vi "Seq Dialog Check RSLinx Tag Boolean.vi"(8 "Segment Data":T3) -> (0 "Step Hisitory":string[](array[string]), 2 "Segment Data 2":T3)   [LabVIEW 2018]
uses:
  type defs/plc path and tag.ctl
  <vilib>/Platform/dataskt.llb/DataSocket Reference Type.ctl
  type defs/Sequence Info.ctl
  type defs/RSLinx Boolean Cluster.ctl
panel:
  in  "Continue on Fail for Red Rabbit":bool
  in  "timeout (ms)":i32=10000
  in  "Error No.":u16=159
  in  "Boolean":bool
  in  "Tag String":T1={"Tag Name"="S060.PXI.Signals.PlltData.SN", "Network Path"="172.15.51.1,1,0", "use opc"=FALSE, "DataSocket Reference"={"CWDSLib._DCWDataSocket"=refnum, "CWDSLib._DCWData"=refnum, "OnDataUpdated"=0, "OnStatusUpdated"=0}} {"DataSocket Reference"."OnStatusUpdated" format="%.0x"; "DataSocket Reference"."OnDataUpdated" format="%.0x"}
  out "Name":string="Pre Run Station - Glass - Vent Open"
  in  "Description":string
  in  "Save":bool
  in  "Cancel":bool
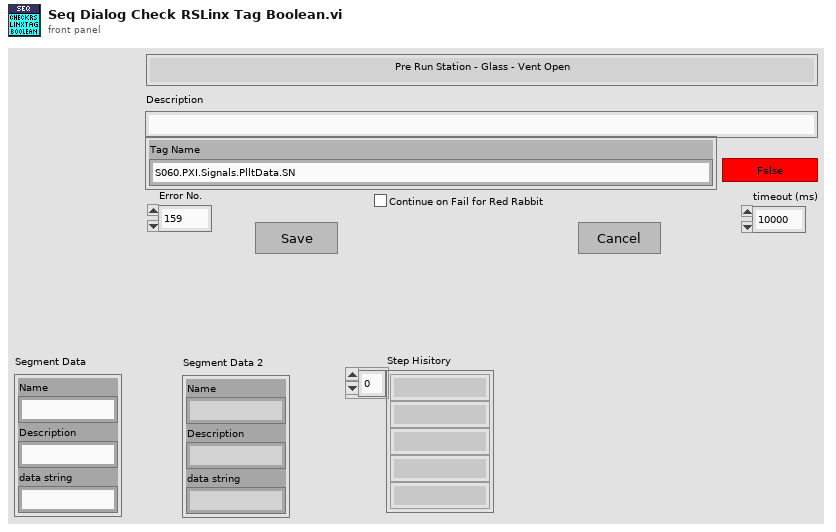
[diagram p1: front panel]
types:
  T1 = typedef "plc path and tag.ctl" = cluster{"Tag Name":string, "Network Path":string, "use opc":bool, "DataSocket Reference":T2}
  T2 = typedef "DataSocket Reference Type.ctl" = cluster{"CWDSLib._DCWDataSocket":refnum<k7>, "CWDSLib._DCWData":refnum<k7>, "OnDataUpdated":u32, "OnStatusUpdated":u32}
  T3 = typedef "Sequence Info.ctl" = cluster{"Name":string, "Description":string, "data string":string}
  T4 = typedef "RSLinx Boolean Cluster.ctl" = cluster{"Data Boolean":bool, "PLC Path and Tag":T1, "Error No.":u16, "timeout (ms)":i32, "Continue on Fail for Red-Rabbit":bool}
  T5 = cluster{"Segment Data":T3, "Old Data":string, "New Data":string, "RSLinx String Cluster":T4}
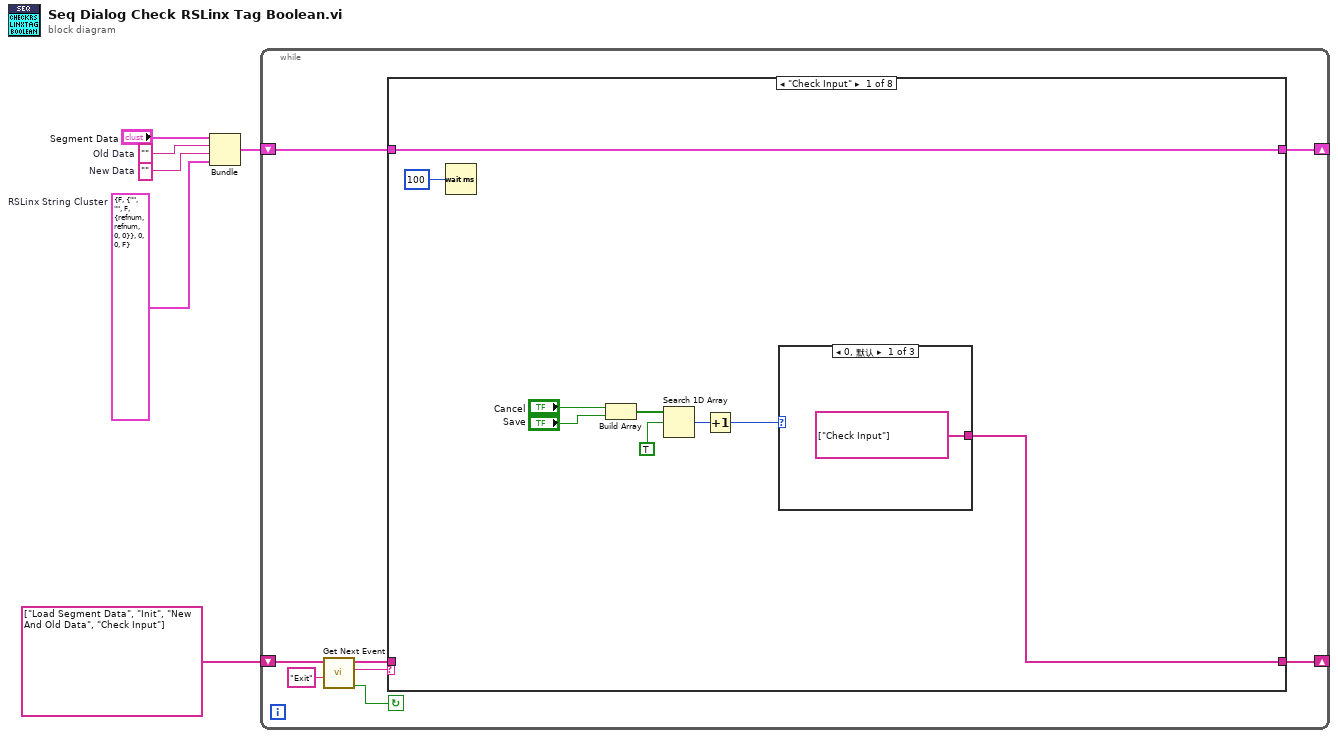
[diagram p0: block diagram]
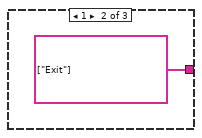
[diagram p2: hidden frame]
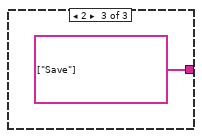
[diagram p3: hidden frame]
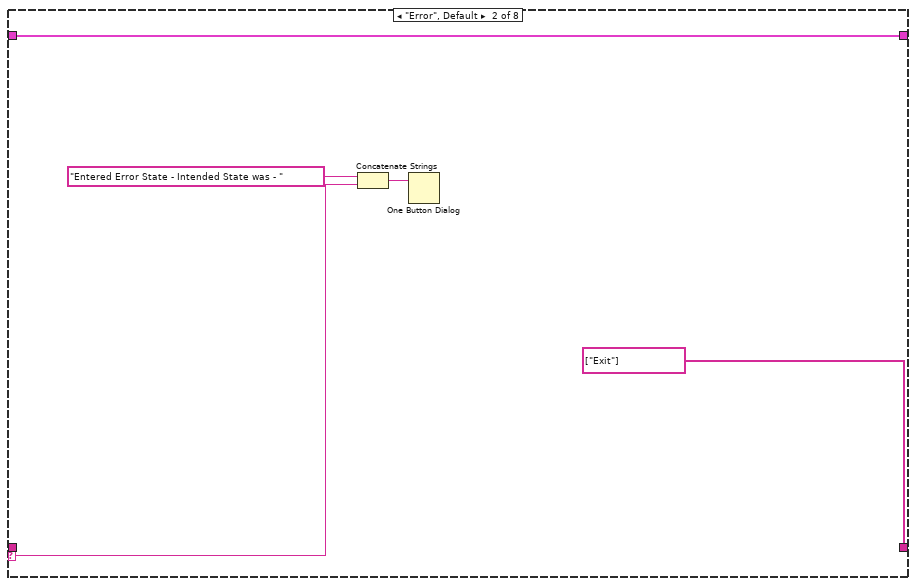
[diagram p4: hidden frame]
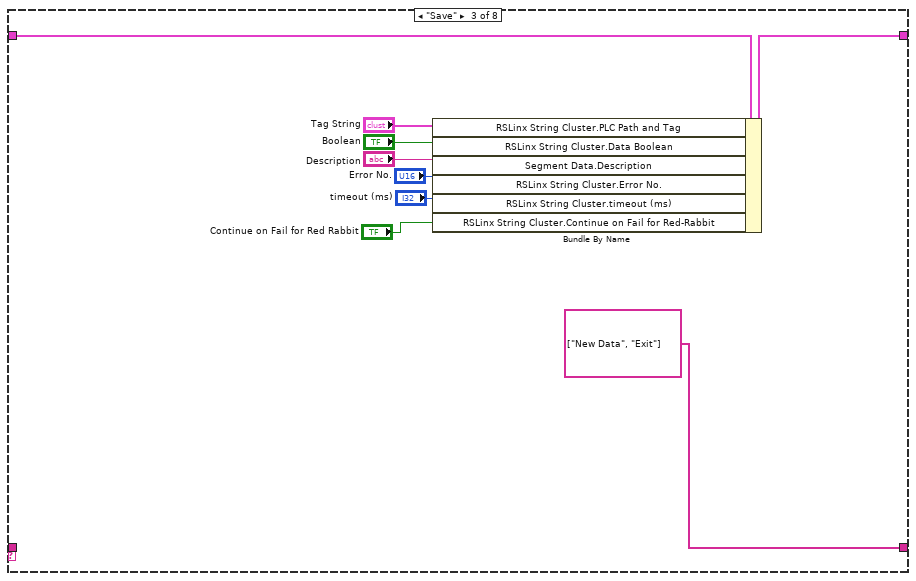
[diagram p5: hidden frame]
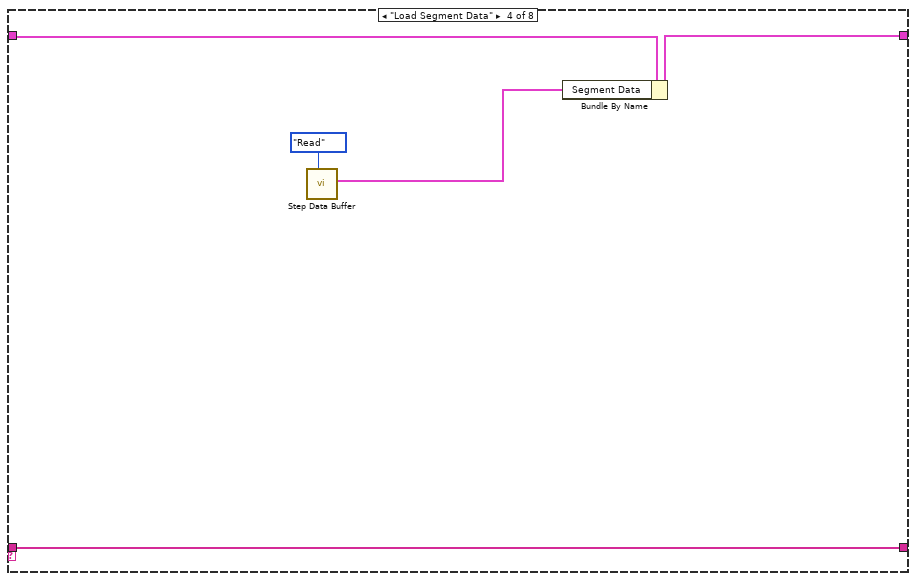
[diagram p6: hidden frame]
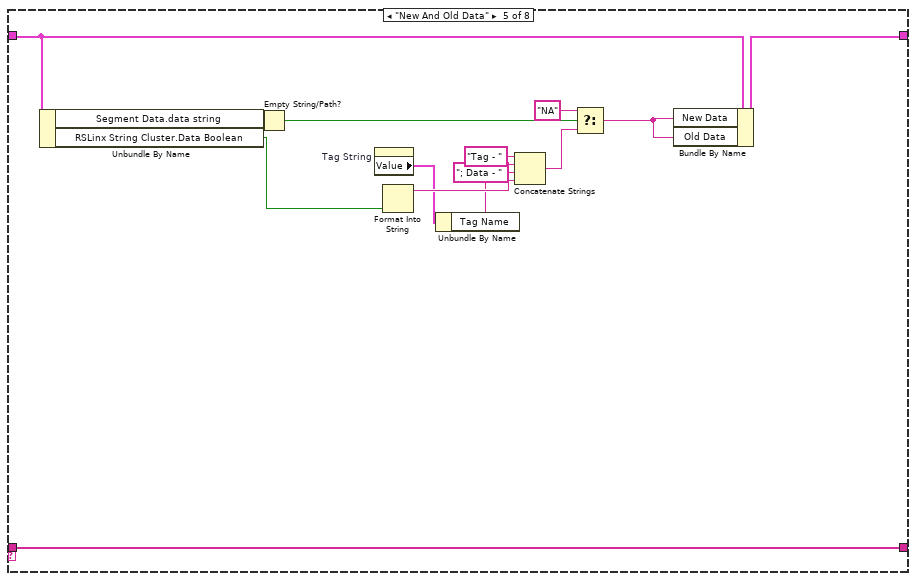
[diagram p7: hidden frame]
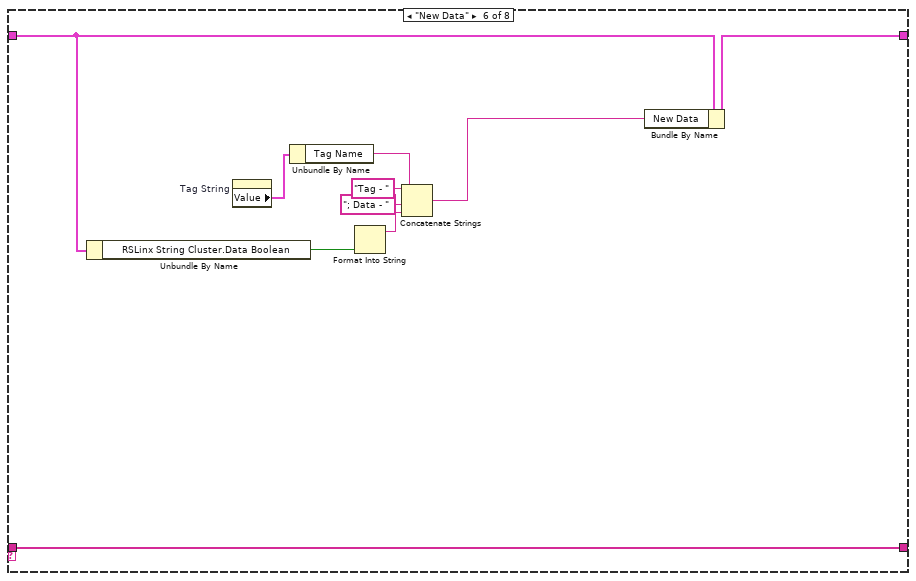
[diagram p8: hidden frame]
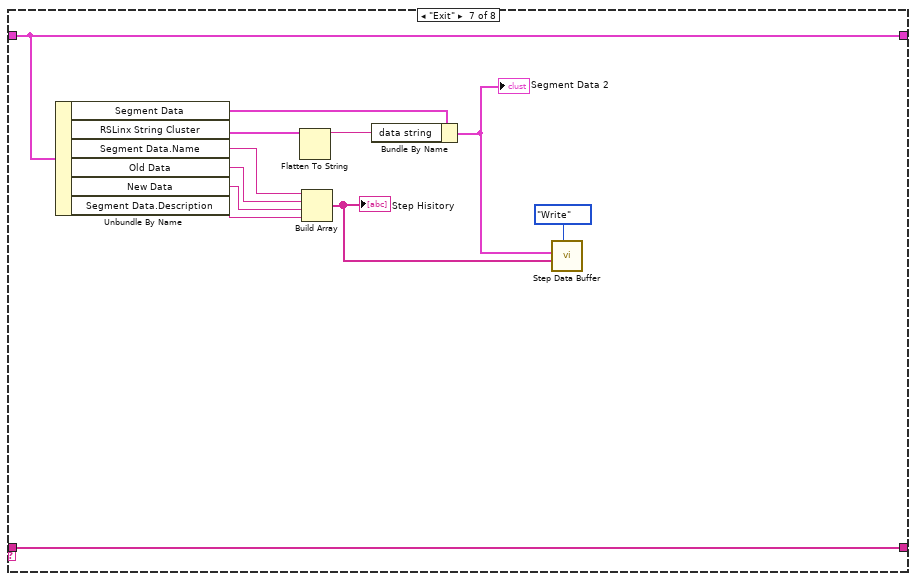
[diagram p9: hidden frame]
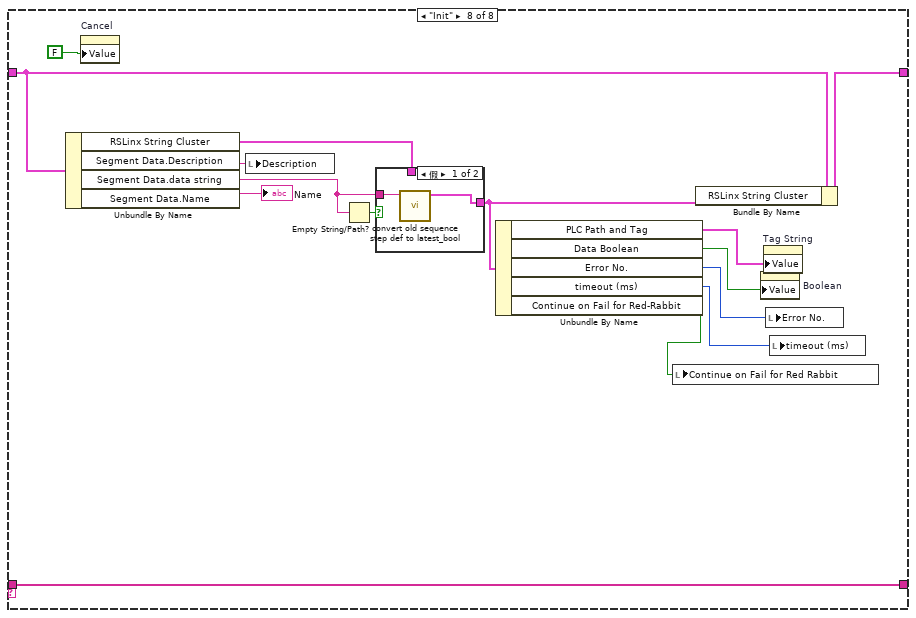
[diagram p10: hidden frame]
diagram:
  w1 = T4 {"Data Boolean"=FALSE, "PLC Path and Tag"={"Tag Name"="", "Network Path"="", "use opc"=FALSE, "DataSocket Reference"={"CWDSLib._DCWDataSocket"=refnum, "CWDSLib._DCWData"=refnum, "OnDataUpdated"=0, "OnStatusUpdated"=0}}, "Error No."=0, "timeout (ms)"=0, "Continue on Fail for Red-Rabbit"=FALSE}  # RSLinx String Cluster
  w3 = ""  # New Data
  w4 = ""  # Old Data
  n1 = Bundle("Segment Data"="Segment Data", "Old Data"=w4, "New Data"=w3, "RSLinx String Cluster"=w1) -> (w6:T5)  [unwired: 1 in]
  n2 = while {
    shift-right: [w12] -> _
    shift-left: string[] ["Load Segment Data", "Init", "New And Old Data", "Check Input"] ("Event queue out") -> [w11]
    shift-right: [w7] -> _
    shift-left: w6 -> [w8]
    stop <- w10 continue-if-true
    n3 = call "Get Next Event.vi"("Exit Event"="Exit", "event queue in"=w11) -> ("Condition (Exit:F)"=w10:bool, "next event"=w14:string, "event queue out"=w13:string[])  [unwired: 3 in]
    n4 = case shown="\"Check Input\"" w14 {
      selector: w14 -> [_ w29 _ _ _ _ _ _]
      tunnel: w13 -> [_ _ _ w41 w53 w69 w81 w96]
      tunnel: [w17 string[] ["Exit"] ("event queue out") string[] ["New Data", "Exit"] ("Event queue out") w41 w53 w69 w81 w96] -> w12
      tunnel: w8 -> [w22 w27 w39 w43 w55 w68 w80 w92]
      tunnel: [w22 w27 w40 w42 w54 w67 w80 w89] -> w7
      frame "Check Input" {
        n5 = Wait (ms)(milliseconds to wait=u32 100) -> ()  [unwired: 1 out]
        n6 = Build Array("Cancel", "Save") -> (w19:bool[])
        n7 = Search 1D Array(1D array=w19, element=TRUE) -> (index of element=w20:i32)  [unwired: 1 in]
        n8 = Increment(x=w20) -> (x+1=w21:i32)
        n9 = case shown="0, 默认" w21 {
          tunnel: [string[] ["Check Input"] ("Events to Insert") string[] ["Exit"] ("Events to Insert") string[] ["Save"] ("Events to Insert")] -> w17
          frame 0, Default {
          }
          frame 1 {
          }
          frame 2 {
          }
        }
      }
      frame "Error", Default {
        n10 = Concatenate Strings("Entered Error State - Intended State was - " ("string"), w29) -> (w31:string)
        n11 = One Button Dialog(message=w31) -> ()  [unwired: 1 in, 1 out]
      }
      frame "Save" {
        n12 = Bundle By Name(cluster=w39, "RSLinx String Cluster.PLC Path and Tag"="Tag String", "RSLinx String Cluster.Data Boolean"="Boolean", "Segment Data.Description"="Description", "RSLinx String Cluster.Error No."="Error No.", "RSLinx String Cluster.timeout (ms)"="timeout (ms)", "RSLinx String Cluster.Continue on Fail for Red-Rabbit"="Continue on Fail for Red Rabbit") -> (w40:T5)
      }
      frame "Load Segment Data" {
        n13 = call "Step Data Buffer.vi"("Mode"=enum16{"Init", "Read", "Write"}."Read") -> ("Segment Data Out"=w45:T3)  [unwired: 6 in, 4 out]
        n14 = Bundle By Name(cluster=w43, "Segment Data"=w45) -> (w42:T5)
      }
      frame "New And Old Data" {
        n15 = Unbundle By Name(w55) -> ("Segment Data.data string"=w59:string, "RSLinx String Cluster.Data Boolean"=w49:bool)
        n16 = Empty String/Path?(string/path=w59) -> (empty?=w56:bool)
        n17 = property on="Tag String" class="Clust (严格)"() -> ("Value"=w47:T1)  [unwired: 2 in, 2 out]
        n18 = Format Into String(w49) -> (resulting string=w48:string)  [unwired: 3 in, 1 out]
        n19 = Unbundle By Name(w47) -> ("Tag Name"=w46:string)
        n20 = Concatenate Strings("Tag - " ("string"), w46, "; Data - " ("string"), w48) -> (w50:string)
        n21 = Select(t="NA", s=w56, f=w50) -> (s? t:f=w58:string)
        n22 = Bundle By Name(cluster=w55, "New Data"=w58, "Old Data"=w58) -> (w54:T5)
      }
      frame "New Data" {
        n23 = Unbundle By Name(w68) -> ("RSLinx String Cluster.Data Boolean"=w63:bool)
        n24 = property on="Tag String" class="Clust (严格)"() -> ("Value"=w61:T1)  [unwired: 2 in, 2 out]
        n25 = Unbundle By Name(w61) -> ("Tag Name"=w60:string)
        n26 = Format Into String(w63) -> (resulting string=w62:string)  [unwired: 3 in, 1 out]
        n27 = Concatenate Strings("Tag - " ("string"), w60, "; Data - " ("string"), w62) -> (w64:string)
        n28 = Bundle By Name(cluster=w68, "New Data"=w64) -> (w67:T5)
      }
      frame "Exit" {
        n29 = Unbundle By Name(w80) -> ("Segment Data"=w73:T3, "RSLinx String Cluster"=w71:T4, "Segment Data.Name"=w79:string, "Old Data"=w78:string, "New Data"=w77:string, "Segment Data.Description"=w74:string)
        n30 = Flatten To String(anything=w71) -> (data string=w70:string)  [unwired: 3 in, 2 out]
        n31 = Build Array(w79, w78, w77, w74) -> (w75:string[])
        "Step Hisitory" <- w75
        n32 = Bundle By Name(cluster=w73, "data string"=w70) -> (w72:T3)
        "Segment Data 2" <- w72
        n33 = call "Step Data Buffer.vi"("Mode"=enum16{"Init", "Read", "Write"}."Write", "Step Hisitory In"=w75, "Segment Data In"=w72) -> ()  [unwired: 4 in, 5 out]
      }
      frame "Init" {
        n34 = Unbundle By Name(w92) -> ("RSLinx String Cluster"=w86:T4, "Segment Data.Description"=w95:string, "Segment Data.data string"=w90:string, "Segment Data.Name"=→"Name":string)
        n35 = property on="Cancel" class="Bool (严格)"("Value"=FALSE ("Cancel")) -> ()  [unwired: 2 in, 2 out]
        n36 = local write "Description"(w95) -> ()
        n37 = Empty String/Path?(string/path=w90) -> (empty?=w91:bool)
        n38 = case shown="假" w91 {
          tunnel: w90 -> [w97 _]
          tunnel: w86 -> [_ w99]
          tunnel: [w98 w99] -> w85
          frame False {
            n39 = call "convert old sequence step def to latest_bool.vi"("data string"=w97) -> ("RSLinx String Cluster out"=w98:T4)  [unwired: 9 in, 1 out]
          }
          frame True {
          }
        }
        n40 = Unbundle By Name(w85) -> ("PLC Path and Tag"=w88:T1, "Data Boolean"=w87:bool, "Error No."=w84:u16, "timeout (ms)"=w83:i32, "Continue on Fail for Red-Rabbit"=w82:bool)
        n41 = local write "Continue on Fail for Red Rabbit"(w82) -> ()
        n42 = Bundle By Name(cluster=w92, "RSLinx String Cluster"=w85) -> (w89:T5)
        n43 = property on="Boolean" class="Bool (严格)"("Value"=w87) -> ()  [unwired: 2 in, 2 out]
        n44 = property on="Tag String" class="Clust (严格)"("Value"=w88) -> ()  [unwired: 2 in, 2 out]
        n45 = local write "Error No."(w84) -> ()
        n46 = local write "timeout (ms)"(w83) -> ()
      }
    }
  }
